vi "update DI and DO.vi"(8 "error in (no error)":errorcluster, 9 "Value":dbl, 10 "DO tasks":refnum<k21>, 11 "Refnum in":refnum<k21>) -> (0 "error out":errorcluster)   [LabVIEW 2020, in "DaqPad_NI6009.lvclass"]
uses:
  DaqPad_NI6009.lvclass
  OnOffTypeDef.ctl
  DAQmx Fill In Error Info.vi
  <resource>/objmgr/daqmx.rc
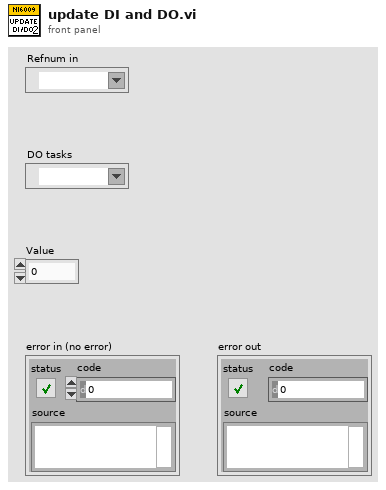
[diagram p1: front panel]
types:
  T1 = typedef "OnOffTypeDef.ctl" = enum16{"off", "on"}
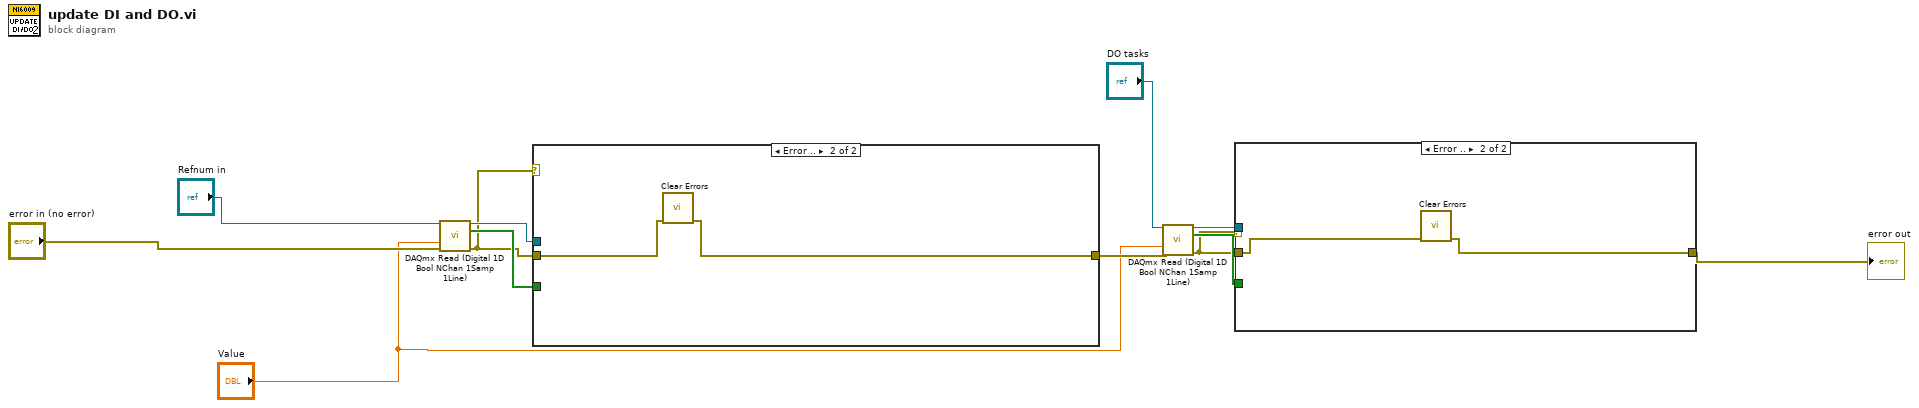
[diagram p0: block diagram]
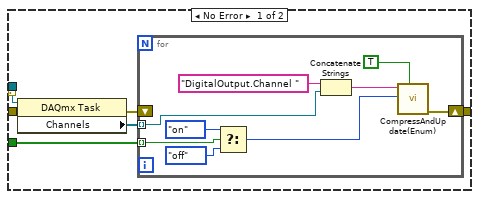
[diagram p2: hidden frame]
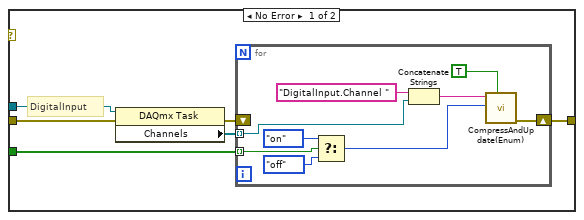
[diagram p3: hidden frame]
diagram:
  n1 = call "DAQmx Read (Digital 1D Bool NChan 1Samp 1Line).vi"("task/channels in"="Refnum in", "timeout"="Value", "error in"="error in (no error)") -> ("task out"=w5:refnum<k21>, "data"=w9:bool[], "error out"=w3:errorcluster)  [unwired: 10 in]
  n2 = case shown="Error .." w3 {
    tunnel: [w18 w28] -> w11
    tunnel: w9 -> [w16 _]
    tunnel: w3 -> [w14 w29]
    tunnel: w5 -> [w13 _]
    frame No Error {
      # "DigitalInput"
      n3 = property class="DAQmx Task"(reference=w13, error in=w14) -> (error out=w17:errorcluster, "Channels"=w15:refnum<k21>[])  [unwired: 1 out]
      n4 = for {
        tunnel: w15 -> [w26] mode=indexing
        tunnel: w16 -> [w23] mode=indexing
        shift-right: [w19] -> w18
        shift-left: w17 -> [_]
        n5 = Select(t=OnOffTypeDef."on" ("Channel 0"), s=w23, f=OnOffTypeDef."off" ("Channel 0")) -> (s? t:f=w20:T1)
        n6 = Concatenate Strings("DigitalInput.Channel " ("string"), w26) -> (w25:string)
        n7 = call "CompressAndUpdate(Enum).vi"("force CVT update (false)"=TRUE, "enum variant"=w20, "command or variable name"=w25) -> ("error out"=w19:errorcluster)  [unwired: 8 in]
      }
    }
    frame Error {
      n8 = call "Clear Errors.vi"("error in (no error)"=w29) -> ("error out"=w28:errorcluster)  [unwired: 5 in, 1 out]
    }
  }
  n9 = call "DAQmx Read (Digital 1D Bool NChan 1Samp 1Line).vi"("task/channels in"="DO tasks", "timeout"="Value", "error in"=w11) -> ("task out"=w8:refnum<k21>, "data"=w10:bool[], "error out"=w2:errorcluster)  [unwired: 10 in]
  n10 = case shown="Error .." w2 {
    tunnel: w10 -> [w33 _]
    tunnel: w2 -> [w31 w46]
    tunnel: w8 -> [w30 _]
    tunnel: [w35 w45] -> w1
    frame No Error {
      n11 = property class="DAQmx Task"(reference=w30, error in=w31) -> (error out=w34:errorcluster, "Channels"=w32:refnum<k21>[])  [unwired: 1 out]
      n12 = for {
        tunnel: w32 -> [w43] mode=indexing
        tunnel: w33 -> [w40] mode=indexing
        shift-right: [w36] -> w35
        shift-left: w34 -> [_]
        n13 = Select(t=OnOffTypeDef."on" ("Channel 0"), s=w40, f=OnOffTypeDef."off" ("Channel 0")) -> (s? t:f=w37:T1)
        n14 = Concatenate Strings("DigitalOutput.Channel " ("string"), w43) -> (w42:string)
        n15 = call "CompressAndUpdate(Enum).vi"("force CVT update (false)"=TRUE, "enum variant"=w37, "command or variable name"=w42) -> ("error out"=w36:errorcluster)  [unwired: 8 in]
      }
    }
    frame Error {
      n16 = call "Clear Errors.vi"("error in (no error)"=w46) -> ("error out"=w45:errorcluster)  [unwired: 5 in, 1 out]
    }
  }
  "error out" <- w1
